vi "单例模式DEMO(Receiver).vi"() -> ()   [LabVIEW 2013]
uses:
  Single_class/Single.lvclass
  <vilib>/addons/_AddQ/G#Object/G#Object.lvclass
panel:
  out "波形图表":dbl(graph)
  out "# of objects killed":i32
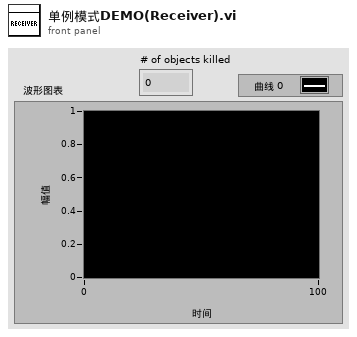
[diagram p1: front panel]
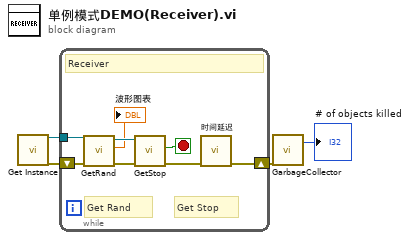
[diagram p0: block diagram]
diagram:
  n1 = call "Get Instance.vi"() -> ("reference out"=w3:refnum<class "Single.lvclass">, "error out"=w4:errorcluster)  [unwired: 18 in]
  n2 = while {
    shift-right: [w12] -> w2
    shift-left: w4 -> [w10]
    tunnel: w3 -> [w11]
    stop <- w7 stop-if-true
    # "Get Stop"
    # "Get Rand"
    # "Receiver"
    n3 = call "GetRand.vi"("error in (no error)"=w10, "reference in"=w11) -> ("error out"=w9:errorcluster, "Rand"=→"波形图表":dbl, "reference out"=w8:refnum<class "Single.lvclass">)  [unwired: 7 in]
    n4 = call-dynamic "GetStop.vi"("error in (no error)"=w9, "reference in"=w8) -> ("error out"=w6:errorcluster, "Stop"=w7:bool)  [unwired: 7 in, 1 out]
    n5 = call "时间延迟"("error in (no error)"=w6) -> ("error out"=w12:errorcluster)  [unwired: 10 in]
  }
  n6 = call <vilib>:"GarbageCollector.vi"("error in (no error)"=w2) -> ("# of objects killed"=→"# of objects killed":i32)  [unwired: 16 in, 2 out]
